vi "GT_SetPos.vi"(3 "pos":i32, 4 "Axis":T1=1 items=["Axis Control"=0, "Axis 1"=1, "Axis 2"=2, "Axis 3"=3, "Axis 4"=4, "Axis 5"=5, "Axis 6"=6, "Axis 7"=7, "Axis 8"=8, "Vector Space Control"=16, "Vector Space 1"=17, "Vector Space 2"=18, "Vector Space 3"=19, "Vector Space 4"=20], 5 "rtn_In":cluster{"rtn":i16, "Func":string}) -> (1 "Axis out":T1=1 items=["Axis Control"=0, "Axis 1"=1, "Axis 2"=2, "Axis 3"=3, "Axis 4"=4, "Axis 5"=5, "Axis 6"=6, "Axis 7"=7, "Axis 8"=8, "Vector Space Control"=16, "Vector Space 1"=17, "Vector Space 2"=18, "Vector Space 3"=19, "Vector Space 4"=20], 2 "rtn_Out":cluster{"rtn":i16, "Func":string})   [LabVIEW 2014]
uses:
  <vilib>/Motion/FlexMotion/CustomControls/CustomControls.llb/AxisOrVectorSpaceControl To Control.flx
  VC6/gts.dll
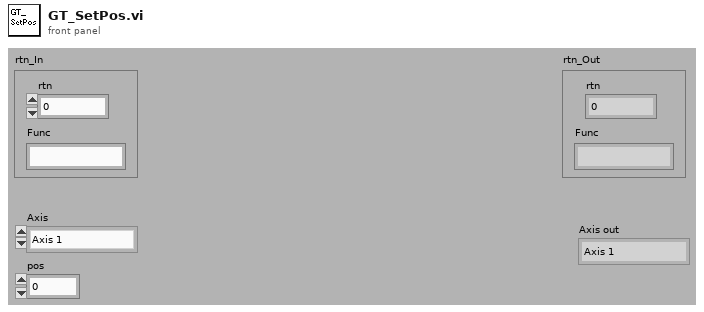
[diagram p1: front panel]
types:
  T1 = typedef "AxisOrVectorSpaceControl To Control.flx" = u16
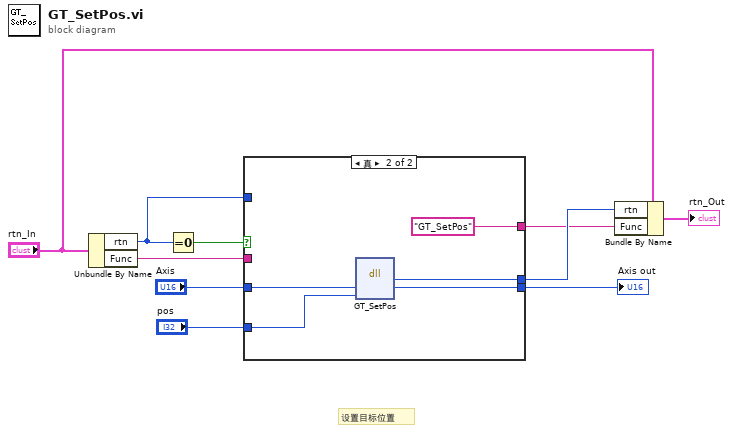
[diagram p0: block diagram]
diagram:
  # "设置目标位置"
  n1 = Unbundle By Name("rtn_In") -> ("rtn"=w5:i16, "Func"=w4:string)
  n2 = Equal To 0?(x=w5) -> (x = 0?=w10:bool)
  n3 = case shown="真" w10 {
    tunnel: [w13 w18] -> w7
    tunnel: [w12 "GT_SetPos" ("Func")] -> w6
    tunnel: w5 -> [w13 _]
    tunnel: w4 -> [w12 _]
    tunnel: "Axis" -> [w11 w16]
    tunnel: "pos" -> [_ w15]
    tunnel: [w11 w14] -> w1
    frame False {
    }
    frame True {
      n4 = dll-call lib="PTH2Fabs DNewGTS AC-800LWin7版源程序-20170926gts85VC6gts.dll" fn="GT_SetPos"("profile"=w16, "pos"=w15) -> ("rtn"=w18:i16, "profile"=w14:i16)  [unwired: 4 in, 2 out]
    }
  }
  "Axis out" <- w1
  n5 = Bundle By Name(cluster="rtn_In", "rtn"=w7, "Func"=w6) -> (→"rtn_Out":cluster{"rtn":i16, "Func":string})
